vi "Find Targeted PPL File Path.vi"(8 "error in (no error)":errorcluster, 9 "Class Name":string, 10 "PPLs Folder Path":path, 11 "Configuration in":refnum<class "Configuration.lvclass">) -> (0 "error out":errorcluster, 2 "PPL File Path":path, 3 "Configuration out":refnum<class "Configuration.lvclass">)   [LabVIEW 2018, in "Configuration.lvlib" / "Configuration.lvclass"]
uses:
  Configuration.lvclass
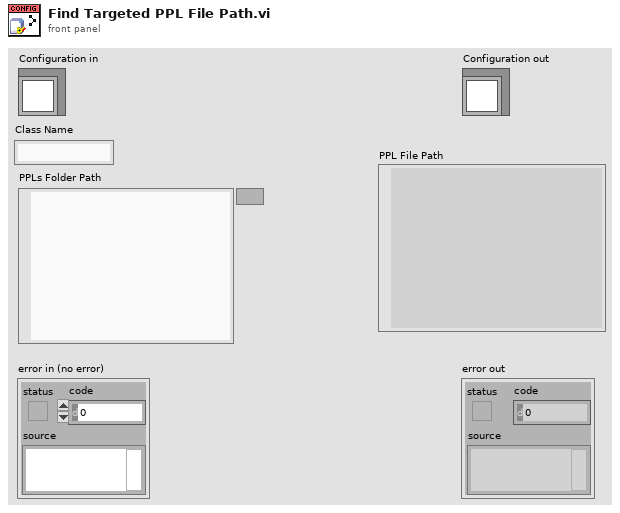
[diagram p1: front panel]
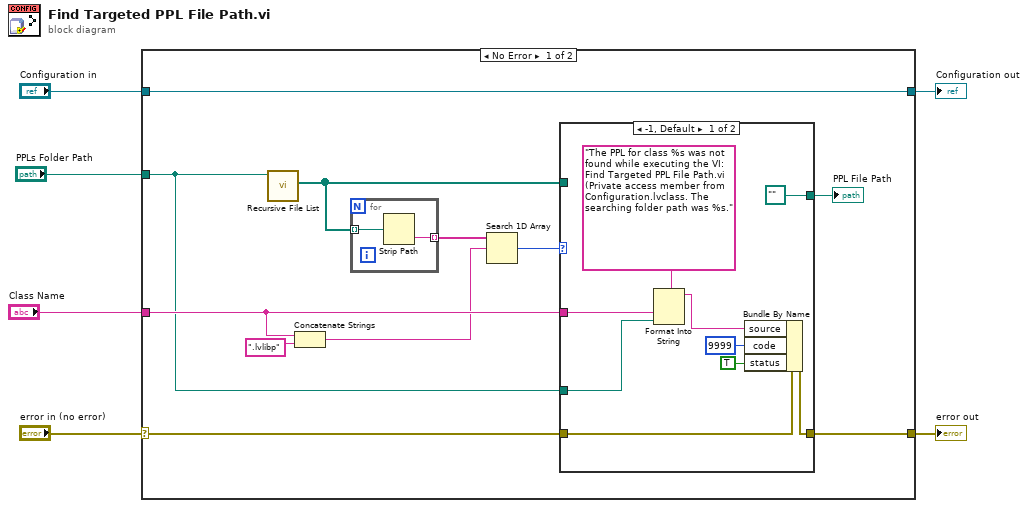
[diagram p0: block diagram]
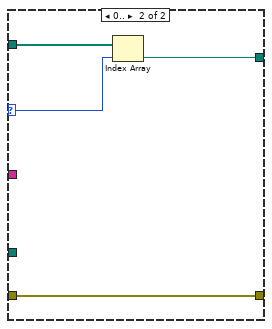
[diagram p2: hidden frame]
diagram:
  n1 = case shown="No Error" "error in (no error)" {
    selector: "error in (no error)" -> [w14 w34]
    tunnel: [w13 w34] -> w5
    tunnel: [w17 w33] -> w3
    tunnel: "Configuration in" -> [w17 w33]
    tunnel: "PPLs Folder Path" -> [w11 _]
    tunnel: "Class Name" -> [w12 _]
    frame No Error {
      n2 = call <vilib>:"Recursive File List.vi"("Folder Path"=w11) -> ("All Files in Dir"=w10:path[])  [unwired: 6 in, 4 out]
      n3 = Concatenate Strings(w12, ".lvlibp" ("string")) -> (w8:string)
      n4 = for {
        tunnel: w10 -> [w19] mode=indexing
        tunnel: [w18] -> w9 mode=indexing
        n5 = Strip Path(path=w19) -> (name=w18:string)  [unwired: 1 out]
      }
      n6 = Search 1D Array(1D array=w9, element=w8) -> (index of element=w7:i32)  [unwired: 1 in]
      n7 = case shown="-1, Default" w7 {
        selector: w7 -> [_ w31]
        tunnel: w10 -> [_ w32]
        tunnel: [path "" w30] -> w15
        tunnel: w14 -> [w27 w29]
        tunnel: [w26 w29] -> w13
        tunnel: w12 -> [w22 _]
        tunnel: w11 -> [w21 _]
        frame -1, Default {
          n8 = Format Into String(format string="The PPL for class %s was not found while executing the VI: Find Targeted PPL File Path.vi (Private access member from Configuration.lvclass. The searching folder path was %s." ("source"), w22, w21) -> (resulting string=w20:string)  [unwired: 2 in, 1 out]
          n9 = Bundle By Name(cluster=w27, "source"=w20, "code"=9999, "status"=TRUE) -> (w26:errorcluster)
        }
        frame 0.. {
          n10 = Index Array(array=w32, index=w31) -> (element=w30:path)
        }
      }
      "PPL File Path" <- w15
    }
    frame Error {
    }
  }
  "error out" <- w5
  "Configuration out" <- w3
